vi "ble_delete_bonding_by_handler.vi"(8 "error in (no error)":errorcluster, 11 "COM Bluegiga in":refnum<visa-resource-name>) -> (0 "error out":errorcluster, 3 "COM Bluegiga out":refnum<visa-resource-name>)   [LabVIEW 2015]
panel:
  in  "Bonding Handle (0xFF = all)":u8=255 format="%02x"
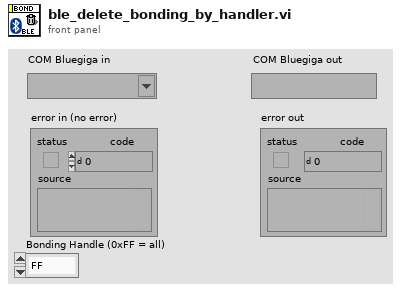
[diagram p1: front panel]
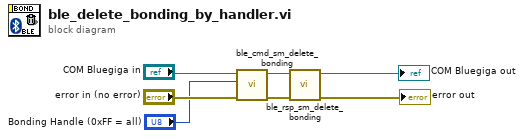
[diagram p0: block diagram]
diagram:
  n1 = call <vilib>:"ble_cmd_sm_delete_bonding.vi"("error in (no error)"="error in (no error)", "Bonding Handle (0xFF = all)"="Bonding Handle (0xFF = all)", "COM Bluegiga in"="COM Bluegiga in") -> ("error out"=w7:errorcluster, "COM Bluegiga out"=w6:refnum<visa-resource-name>)  [unwired: 7 in]
  n2 = call <vilib>:"ble_rsp_sm_delete_bonding.vi"("error in (no error)"=w7, "COM Bluegiga in"=w6) -> ("error out"=→"error out":errorcluster, "COM Bluegiga out"=→"COM Bluegiga out":refnum<visa-resource-name>)  [unwired: 8 in]
